vi "db_learn.vi"() -> ()   [LabVIEW 2011]
uses:
  <vilib>/addons/database/Connection.llb/DB Tools Open Connec (String).vi
  <vilib>/addons/database/Auxilliary.llb/DB Tools Format Datetime String (Time Stamp).vi
  <vilib>/addons/database/NI_Database_API.lvlib
panel:
  in  "sensor1":dbl
  in  "columns":string[](array[string])
  in  "sensor0":dbl
  in  "angle":dbl
  out "date/time string":string
  out "data":variant[][](array[variant])
  out "tables":string[](array[string])
  in  "prompt? (F)":bool
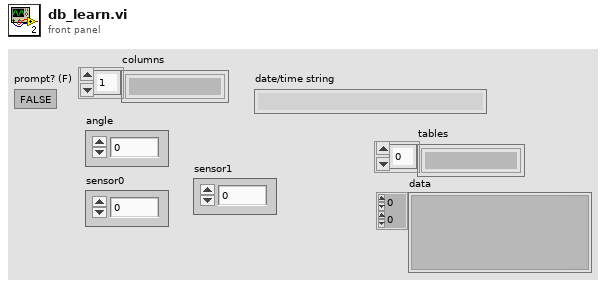
[diagram p1: front panel]
types:
  T1 = cluster{"date/time string":string, "angle":dbl, "sensor0":dbl, "sensor1":dbl}
  T2 = typedef "NI_Database_API.lvlib/Conn ObjectReference.ctl" = refnum<k1>
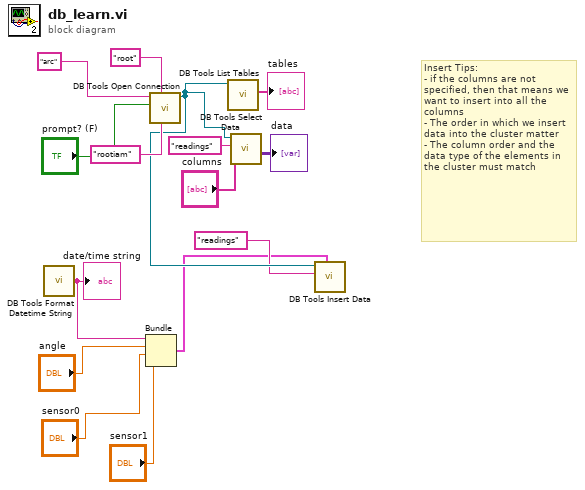
[diagram p0: block diagram]
diagram:
  # "Insert Tips:\n- if the columns are not specified, then that means we want to insert into all the columns\n- The order in which we insert data into the cluster matter\n- The column order and the data type of the elements in the cluster must match"
  n1 = call-poly <vilib>:"DB Tools Format Datetime String.vi"() -> ("date/time string"=w7:string)  [unwired: 1 in]
  "date/time string" <- w7
  n2 = Bundle("date/time string"=w7, "angle"="angle", "sensor0"="sensor0", "sensor1"="sensor1") -> (w4:T1)  [unwired: 1 in]
  n3 = call-poly <vilib>:"DB Tools Open Connection.vi"("password"="rootiam", "userID"="root", "prompt? (F)"="prompt? (F)", "connection information"="arc") -> ("connection reference"=w9:T2)  [unwired: 4 in, 1 out]
  n4 = call <vilib>:"DB Tools List Tables.vi"("connection reference"=w9) -> ("tables"=→"tables":string[])  [unwired: 4 in, 2 out]
  n5 = call <vilib>:"DB Tools Select Data.vi"("columns"="columns", "table"="readings", "connection reference"=w9) -> ("data"=→"data":variant[][])  [unwired: 3 in, 2 out]
  n6 = call <vilib>:"DB Tools Insert Data.vi"("data"=w4, "table"="readings", "connection reference"=w9) -> ()  [unwired: 7 in, 2 out]
